vi "FindNodeByName.vi"(0 "reference":refnum<class "Graph.lvclass">, 1 "Name":string, 5 "error in (no error)":errorcluster) -> (14 "reference out":refnum<class "Graph.lvclass">, 15 "node":refnum<class "AbstractNode.lvclass">, 16 "found":bool, 19 "error out":errorcluster)   [LabVIEW 2012, in "Graph.lvclass"]
doc: "Finds a node containing the given point.\n @param p a point\n @return a node containing p or null if no nodes contain p\n */\n public Node findNode(Point2D p)"
uses:
  <resource>/Framework/Providers/Open_GDS/UML/Graph_class/Graph.lvclass
  <resource>/Framework/Providers/Open_GDS/UML/AbstractNode_class/AbstractNode.lvclass
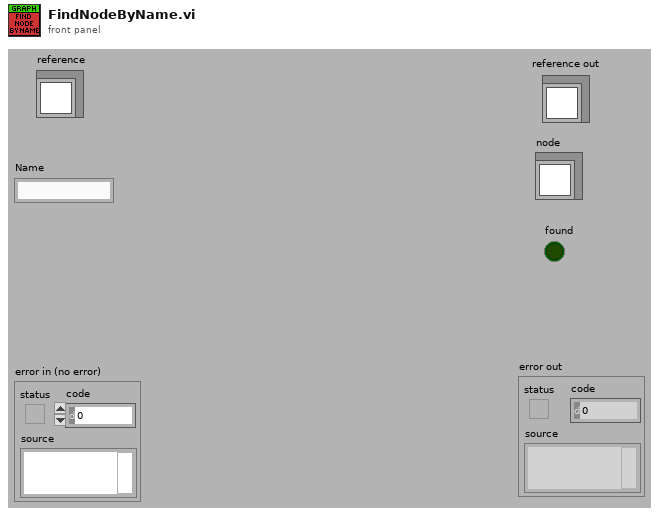
[diagram p1: front panel]
types:
  T1 = typedef "Graph.lvclass/ObjectAttributes.ctl" = cluster{"nodes":refnum<class "AbstractNode.lvclass">[], "edges":refnum<class "AbstractEdge.lvclass">[], "nodesToBeRemoved":refnum<class "AbstractNode.lvclass">[], "edgesToBeRemoved":refnum<class "AbstractEdge.lvclass">[], "needsLayout":bool, "LayoutNodes":refnum<class "AbstractNode.lvclass">[]}
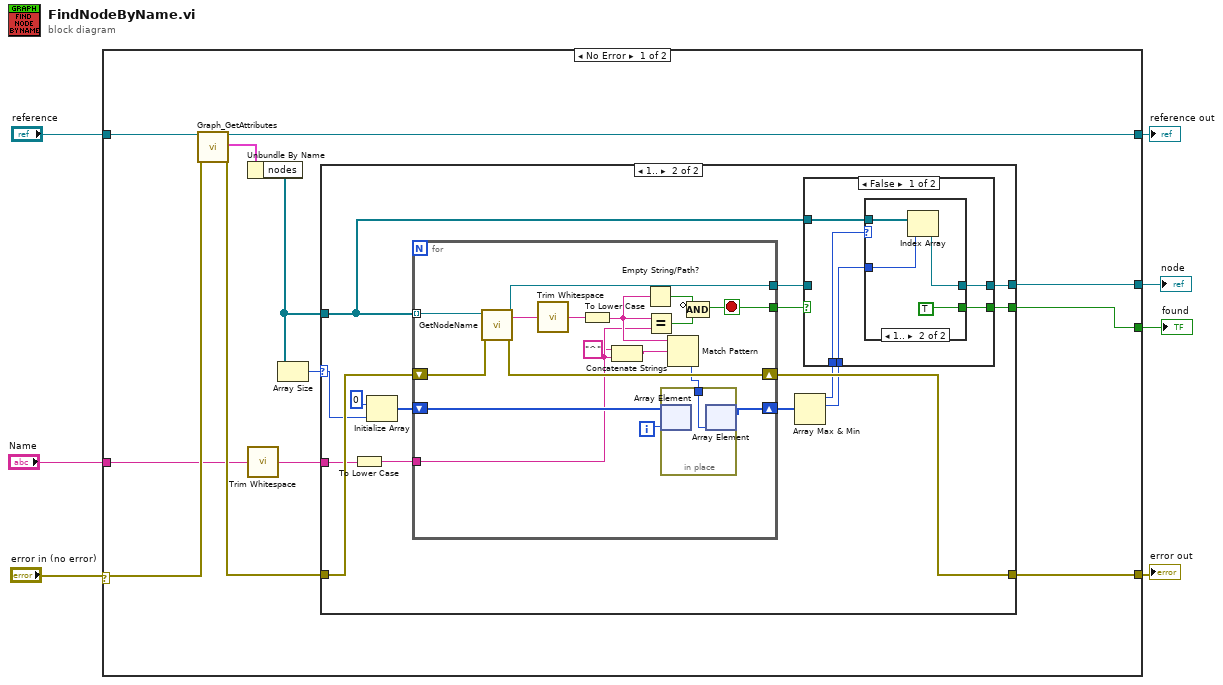
[diagram p0: block diagram]
diagram:
  n1 = case shown="No Error" "error in (no error)" {
    selector: "error in (no error)" -> [w16 w65]
    tunnel: "reference" -> [w19 w66]
    tunnel: [w18 w65] -> w6
    tunnel: [w17 w66] -> w5
    tunnel: [w9 _] -> w3
    tunnel: [w8 _] -> w2
    tunnel: "Name" -> [w11 _]
    frame No Error {
      n2 = call <resource>:"Graph_GetAttributes.vi"("reference in"=w19, "error in (no error)"=w16) -> ("reference out"=w17:refnum<class "Graph.lvclass">, "Attributes"=w15:T1, "error out"=w13:errorcluster)  [unwired: 15 out]
      n3 = Unbundle By Name(w15) -> ("nodes"=w14:refnum<class "AbstractNode.lvclass">[])
      n4 = call <vilib>:"Trim Whitespace.vi"("string"=w11) -> ("trimmed string"=w10:string)  [unwired: 1 in]
      n5 = Array Size(array=w14) -> (size(s)=w12:i32)
      n6 = case shown="1.." w12 {
        selector: w12 -> [_ w30]
        tunnel: w14 -> [_ w23]
        tunnel: w13 -> [w20 w35]
        tunnel: [w20 w34] -> w18
        tunnel: [_ w26] -> w9
        tunnel: w10 -> [_ w33]
        tunnel: [_ w24] -> w8
        frame 0, Default {
        }
        frame 1.. {
          n7 = To Lower Case(string=w33) -> (all lower case string=w32:string)
          n8 = Initialize Array(0 ("offset past match"), w30) -> (w31:i32[])
          n9 = for {
            tunnel: w23 -> [w63] mode=indexing
            shift-right: [w61] -> w34
            shift-left: w35 -> [w62]
            tunnel: w32 -> [w49]
            tunnel: [w55] -> w25
            tunnel: [w58] -> w27
            shift-right: [w50] -> w28
            shift-left: w31 -> [w51]
            i -> [w54]
            stop <- w55 stop-if-true
            n10 = call-dynamic "GetNodeName.vi"("reference in"=w63, "error in (no error)"=w62) -> ("reference out"=w58:refnum<class "AbstractNode.lvclass">, "String"=w60:string, "error out"=w61:errorcluster)  [unwired: 15 in]
            n11 = call <vilib>:"Trim Whitespace.vi"("string"=w60) -> ("trimmed string"=w59:string)  [unwired: 1 in]
            n12 = To Lower Case(string=w59) -> (all lower case string=w53:string)
            n13 = Concatenate Strings("^" ("string"), w49) -> (w48:string)
            n14 = Empty String/Path?(string/path=w53) -> (empty?=w56:bool)
            n15 = Equal?(x=w53, y=w49) -> (x = y?=w57:bool)
            n16 = Match Pattern(string=w53, regular expression=w48) -> (offset past match=w52:i32)  [unwired: 1 in, 3 out]
            n17 = in-place {
              in-place-border: w52 -> [w64]
              n18 = in-place-array #1(w51, w54) -> ()  [unwired: 1 out]
              n19 = in-place-array #1(w64) -> (w50:i32[])  [unwired: 1 out]
            }
            n20 = Compound Arithmetic op=AND(invert w56, w57) -> (w55:bool)
          }
          n21 = Array Max & Min(array=w28) -> (max value=w21:i32, max index (indices)=w22:i32)  [unwired: 2 out]
          n22 = case shown="False" w25 {
            selector: w25 -> [_ w45]
            tunnel: w27 -> [_ w46]
            tunnel: [w39 w46] -> w26
            tunnel: [w38 w45] -> w24
            tunnel: w23 -> [w40 _]
            tunnel: w22 -> [w36 _]
            tunnel: w21 -> [w37 _]
            frame False {
              n23 = case shown="1.." w37 {
                tunnel: w40 -> [_ w44]
                tunnel: [_ w43] -> w39
                tunnel: [_ TRUE] -> w38
                tunnel: w36 -> [_ w41]
                frame 0, Default {
                }
                frame 1.. {
                  n24 = Index Array(array=w44, index=w41) -> (element=w43:refnum<class "AbstractNode.lvclass">)
                }
              }
            }
            frame True {
            }
          }
        }
      }
    }
    frame Error {
    }
  }
  "reference out" <- w5
  "error out" <- w6
  "found" <- w2
  "node" <- w3
